vi "read_channels_specify_range_VISA.vi"(5 "postDAQ  wait ms":u32=12, 7 "preDAQ  wait ms":u32=25, 8 "error in":T1, 10 "range":dbl[](array[numeric])=[3e-05, 2e-09, 3e-05] format="%^#_6g", 11 "VISA resource in":refnum<visa-resource-name>) -> (0 "error out":T1, 2 "data":dbl[](array[numeric]), 3 "VISA resource out":refnum<visa-resource-name>)   [LabVIEW 2024]
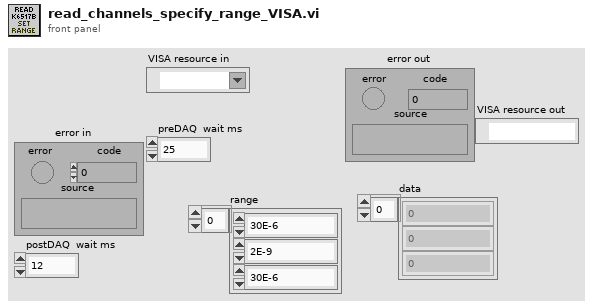
[diagram p1: front panel]
types:
  T1 = cluster{"error":bool, "code":i32, "source":string}
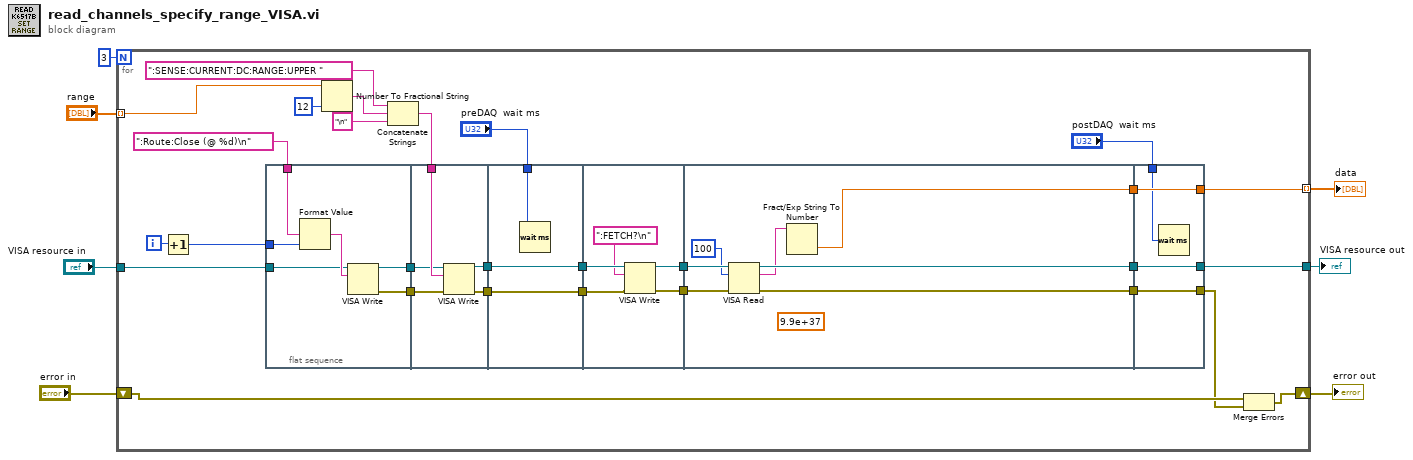
[diagram p0: block diagram]
diagram:
  n1 = for {
    N: 3 -> [_]
    shift-right: [w35] -> w3
    shift-left: "error in" -> [w32]
    tunnel: "range" -> [w27] mode=indexing
    tunnel: [w28] -> w4 mode=indexing
    tunnel: "VISA resource in" -> [w24]
    tunnel: [w16] -> w1
    i -> [w34]
    n2 = Increment(x=w34) -> (x+1=w33:i32)
    n3 = flat-sequence {
      tunnel: w33 -> [w38]
      tunnel: [w39] -> w31
      tunnel: w24 -> [w40]
      tunnel: [w37] -> w21
      tunnel: ":Route:Close (@ %d)\n" -> [w36]
      tunnel: [w45] -> w30
      tunnel: w31 -> [w46]
      tunnel: w22 -> [w44]
      tunnel: w21 -> [w43]
      tunnel: [w42] -> w20
      tunnel: w30 -> [w49]
      tunnel: [w49] -> w29
      tunnel: "preDAQ  wait ms" -> [w48]
      tunnel: w20 -> [w47]
      tunnel: [w47] -> w19
      tunnel: w29 -> [w54]
      tunnel: w19 -> [w53]
      tunnel: [w51] -> w18
      tunnel: [w50] -> w17
      tunnel: [w61] -> w11
      tunnel: [w60] -> w10
      tunnel: [w59] -> w9
      tunnel: w17 -> [w57]
      tunnel: w18 -> [w58]
      tunnel: [w65] -> w28
      tunnel: w11 -> [w65]
      tunnel: "postDAQ  wait ms" -> [w64]
      tunnel: [w63] -> w16
      tunnel: w10 -> [w63]
      tunnel: [w62] -> w12
      tunnel: w9 -> [w62]
      frame #0 {
        n4 = Format Value(format string=w36, value (0)=w38) -> (output string=w41:string)  [unwired: 1 in]
        n5 = VISA Write(VISA resource name=w40, write buffer=w41) -> (VISA resource name out=w37:refnum<visa-resource-name>, error out=w39:errorcluster)  [unwired: 1 in, 1 out]
      }
      frame #1 {
        n6 = VISA Write(VISA resource name=w43, write buffer=w44, error in (no error)=w46) -> (VISA resource name out=w42:refnum<visa-resource-name>, error out=w45:errorcluster)  [unwired: 1 out]
      }
      frame #2 {
        n7 = Wait (ms)(milliseconds to wait=w48) -> ()  [unwired: 1 out]
      }
      frame #3 {
        n8 = VISA Write(VISA resource name=w53, write buffer=":FETCH?\n", error in (no error)=w54) -> (VISA resource name out=w51:refnum<visa-resource-name>, error out=w50:errorcluster)  [unwired: 1 out]
      }
      frame #4 {
        (unwired) 9.9e+37 ("pd2_v")
        n9 = VISA Read(VISA resource name=w58, byte count=u32 100, error in (no error)=w57) -> (VISA resource name out=w60:refnum<visa-resource-name>, read buffer=w55:string, error out=w59:errorcluster)  [unwired: 1 out]
        n10 = Fract/Exp String To Number(string=w55) -> (number=w61:dbl)  [unwired: 3 in, 1 out]
      }
      frame #5 {
        n11 = Wait (ms)(milliseconds to wait=w64) -> ()  [unwired: 1 out]
      }
    }
    n12 = Number To Fractional String(number=w27, precision (6)=i16 12) -> (F-format string=w26:string)  [unwired: 2 in]
    n13 = Concatenate Strings(":SENSE:CURRENT:DC:RANGE:UPPER ", w26, "\n") -> (w22:string)
    n14 = Merge Errors(w32, w12) -> (w35:errorcluster)
  }
  "error out" <- w3
  "data" <- w4
  "VISA resource out" <- w1
